vi "Index.vi"(8 "error in (no error)":errorcluster, 10 "Index":i32, 11 "Path Array in":refnum<class "Path Array.lvclass">) -> (0 "error out":errorcluster, 3 "Indexed element":refnum<class "Generic Data.lvclass">)   [LabVIEW 2020, in "Data.lvlib" / "Path Array.lvclass"]
doc: "Index an element from 'Generic Data in'.\nThis implementation returns a generic String class with the indexed string."
uses:
  Path Array.lvclass
  Generic Data.lvclass
  Path Array.lvclass/Path Array.ctl
  Path/Path.lvclass/Path.ctl
  Path/Path.lvclass
  C:/Users/Henri/OneDrive/LabVIEW/Framework/Data/Generic Data/Generic Data.lvclass
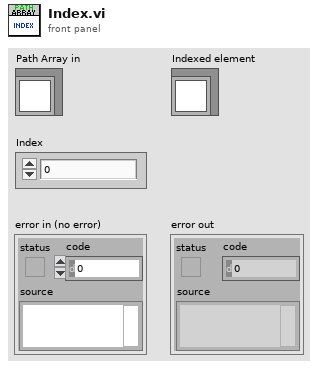
[diagram p1: front panel]
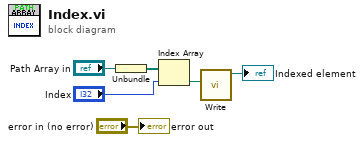
[diagram p0: block diagram]
diagram:
  n1 = Unbundle("Path Array in") -> (w5:path[])
  n2 = Index Array(array=w5, index="Index") -> (element=w2:path)
  n3 = call "Write.vi"("Path"=w2) -> ("Path out"=→"Indexed element":refnum<class "Path.lvclass">)  [unwired: 10 in]
  "error out" <- "error in (no error)"
